vi "STEPSTATE.vi"(0 "VISA resource name":refnum<visa-resource-name>, 11 "error in (no error)":errorcluster) -> (4 "VISA resource name out":refnum<visa-resource-name>, 6 "Test Step State":string="\r\n", 8 "Error Message":string, 10 "Error Code":i32, 15 "error out":errorcluster)   [LabVIEW 2010, in "VITREK V7X.lvlib"]
doc: "Responds with a <String> indicating the pass/fail state of each test step. This can also be used while running a test sequence. The response contains one character for each defined test step,\nP passed\nF failed\n- Not performed\n? in process\n\n<b>Note:</b> please refer to the instrument manual for the <b>STAT?</b> specification."
uses:
  VITREK V7X.lvlib
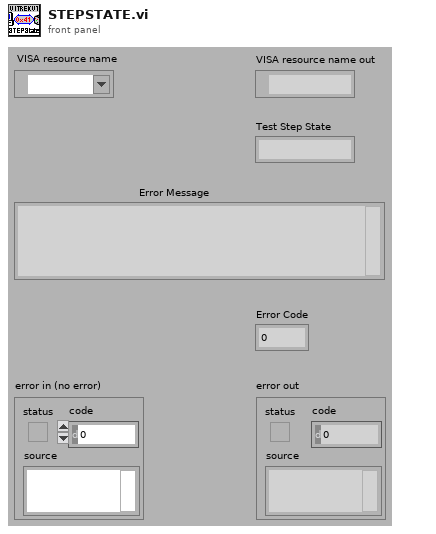
[diagram p1: front panel]
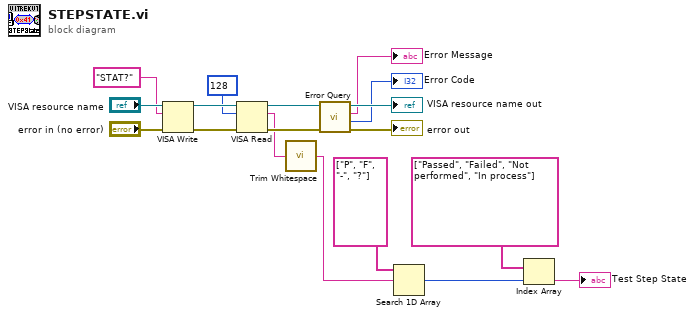
[diagram p0: block diagram]
diagram:
  n1 = VISA Write(VISA resource name="VISA resource name", write buffer="STAT?", error in (no error)="error in (no error)") -> (VISA resource name out=w14:refnum<visa-resource-name>, error out=w12:errorcluster)  [unwired: 1 out]
  n2 = VISA Read(VISA resource name=w14, byte count=u32 128, error in (no error)=w12) -> (VISA resource name out=w13:refnum<visa-resource-name>, read buffer=w8:string, error out=w9:errorcluster)  [unwired: 1 out]
  n3 = call <vilib>:"Trim Whitespace.vi"("string"=w8) -> ("trimmed string"=w2:string)  [unwired: 1 in]
  n4 = call "Error Query.vi"("error in (no error)"=w9, "VISA resource name"=w13) -> ("error out"=→"error out":errorcluster, "Error Code"=→"Error Code":i32, "Error Message"=→"Error Message":string, "VISA resource name out"=→"VISA resource name out":refnum<visa-resource-name>)  [unwired: 6 in]
  n5 = Search 1D Array(1D array=string[] ["P", "F", "-", "?"], element=w2) -> (index of element=w3:i32)  [unwired: 1 in]
  n6 = Index Array(array=string[] ["Passed", "Failed", "Not performed", "In process"], index=w3) -> (element=→"Test Step State":string)
